vi "有问题先运行我保存VI更新依赖.vi"() -> ()   [LabVIEW 2017]
panel:
  out "Path Indicator":path
  out "save":dbl(slide) scale=0.0..1.0
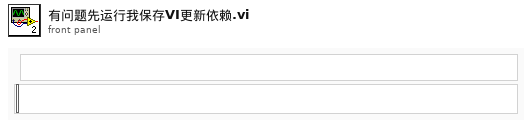
[diagram p1: front panel]
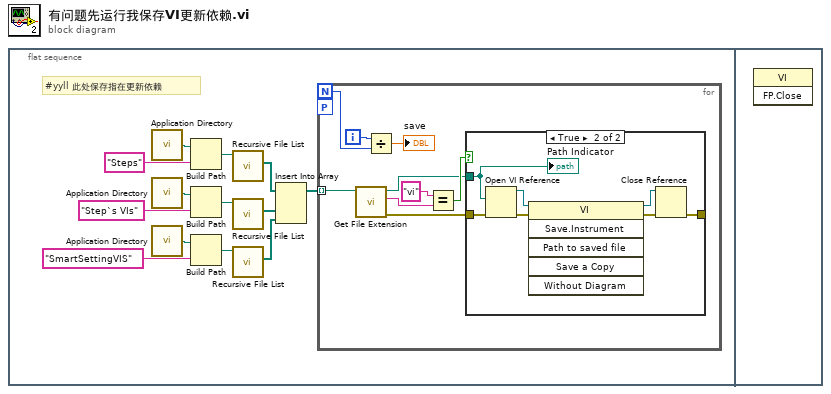
[diagram p0: block diagram]
diagram:
  n1 = flat-sequence {
    frame #0 {
      # "#yyll 此处保存指在更新依赖"
      n2 = call <vilib>:"Application Directory.vi"() -> ("Application Directory"=w12:path)
      n3 = call <vilib>:"Application Directory.vi"() -> ("Application Directory"=w9:path)
      n4 = call <vilib>:"Application Directory.vi"() -> ("Application Directory"=w6:path)
      n5 = Build Path(base path=w12, name or relative path="Steps") -> (appended path=w13:path)
      n6 = Build Path(base path=w9, name or relative path="Step`s VIs") -> (appended path=w8:path)
      n7 = Build Path(base path=w6, name or relative path="SmartSettingVIS") -> (appended path=w7:path)
      n8 = call <vilib>:"Recursive File List.vi"("Folder Path"=w13) -> ("All Files in Dir"=w4:path[])  [unwired: 6 in, 4 out]
      n9 = call <vilib>:"Recursive File List.vi"("Folder Path"=w8) -> ("All Files in Dir"=w3:path[])  [unwired: 6 in, 4 out]
      n10 = call <vilib>:"Recursive File List.vi"("Folder Path"=w7) -> ("All Files in Dir"=w2:path[])  [unwired: 6 in, 4 out]
      n11 = Insert Into Array(array=w4, new element #1=w3, new element #2=w2) -> (w1:path[])  [unwired: 1 in]
      n12 = for {
        N -> [w15]
        tunnel: w1 -> [w20] mode=indexing
        workers-P: _ -> [_]
        i -> [w16]
        n13 = call <vilib>:"Get File Extension.vi"("file"=w20) -> ("error out"=w17:errorcluster, "lowercase file extension"=w22:string, "dup file"=w18:path)  [unwired: 6 in, 2 out]
        n14 = Divide(x=w16, y=w15) -> (x/y=→"save":dbl)
        n15 = Equal?(x="vi", y=w22) -> (x = y?=w19:bool)
        n16 = case shown="True" w19 {
          tunnel: w18 -> [_ w23]
          tunnel: [_ w25] -> _
          tunnel: w17 -> [_ w24]
          frame False {
          }
          frame True {
            n17 = Open VI Reference(vi path=w23, error in (no error)=w24) -> (vi reference=w29:refnum<vi>, error out=w28:errorcluster)  [unwired: 4 in]
            n18 = invoke class="VI" method="Save.Instrument"(reference=w29, error in=w28) -> (reference out=w26:refnum<vi>, error out=w27:errorcluster)  [unwired: 4 in, 4 out]
            n19 = Close Reference(reference=w26, error in (no error)=w27) -> (error out=w25:errorcluster)
            "Path Indicator" <- w23
          }
        }
      }
    }
    frame #1 {
      n20 = invoke class="VI" method="FP.Close"() -> ()  [unwired: 3 in, 3 out]
    }
  }
